vi "chart plotarea set gradient.vi"(8 "error in (no error)":errorcluster, 10 "gradient":T1, 11 "chart":u32) -> (0 "error out":errorcluster, 2 "gradient out":T1)   [LabVIEW 8.6]
doc: "void chart_plotarea_set_gradient(lxw_chart chart, lxw_chart_gradient_fill *gradient);"
uses:
  pending_lvxlsxwriter/xlsxwriter.dll
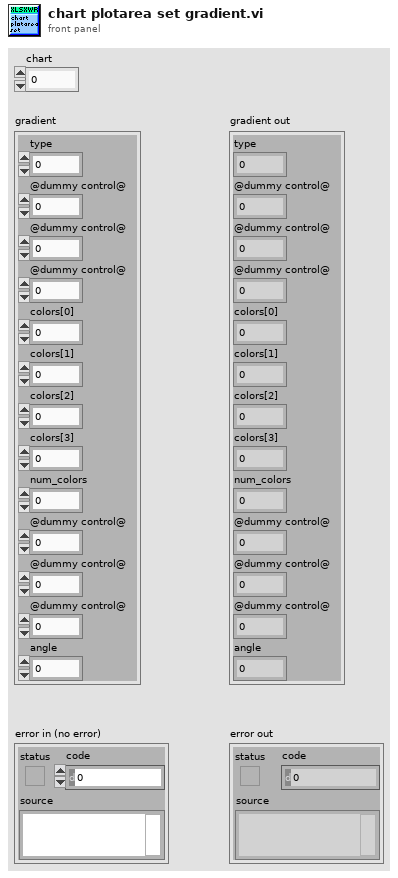
[diagram p1: front panel]
types:
  T1 = cluster{"type":u8, "@dummy control@":i8, "@dummy control@":i8, "@dummy control@":i8, "colors[0]":u32, "colors[1]":u32, "colors[2]":u32, "colors[3]":u32, "num_colors":u8, "@dummy control@":i8, "@dummy control@":i8, "@dummy control@":i8, "angle":dbl}
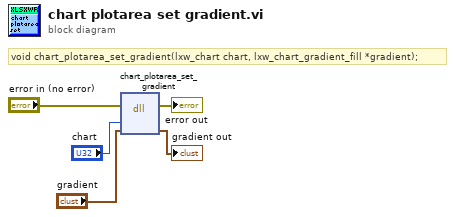
[diagram p0: block diagram]
diagram:
  # "void chart_plotarea_set_gradient(lxw_chart chart, lxw_chart_gradient_fill *gradient);"
  n1 = dll-call lib="C:/Users/WDAGUtilityAccount/Desktop/pending_lvxlsxwriter/xlsxwriter.*" fn="chart_plotarea_set_gradient"(error in="error in (no error)", "chart"="chart", "gradient"="gradient") -> (error out=→"error out":errorcluster, "gradient"=→"gradient out":T1)  [unwired: 4 in, 1 out]
